vi "Next.vi"(7 "Previous In":refnum<class "Known Host.lvclass">, 8 "Error In":errorcluster, 10 "Next In":refnum<class "Known Host.lvclass">, 11 "KnownHosts In":refnum<class "Known Hosts.lvclass">) -> (0 "Error Out":errorcluster, 1 "Result":T1, 2 "Next Out":refnum<class "Known Host.lvclass">, 3 "KnownHosts Out":refnum<class "Known Hosts.lvclass">, 5 "Previous Out":refnum<class "Known Host.lvclass">)   [LabVIEW 2018, in "Toolkit.lvlib" / "Known Hosts.lvclass"]
uses:
  Known Hosts.lvclass
  Known Host/Known Host.lvclass
  Typedefs/Get Results.ctl
  Known Hosts.lvclass/Known Hosts.ctl
  Known Host/Known Host.lvclass/Known Host.ctl
  Session/Session.lvclass/Session.ctl
  SSH/SSH.lvclass/SSH.ctl
  Toolkit.lvlib
  Session/Session.lvclass
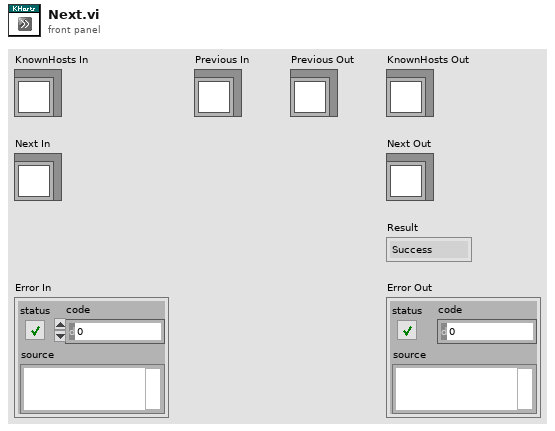
[diagram p1: front panel]
types:
  T1 = typedef "Toolkit.lvlib/Known Hosts.lvclass/Get Results.ctl" = enum32{"Success", "End of Hosts"}
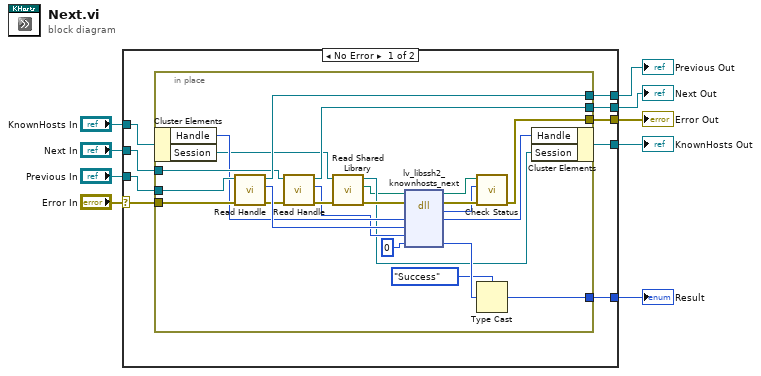
[diagram p0: block diagram]
diagram:
  n1 = case shown="No Error" "Error In" {
    selector: "Error In" -> [w17 w45]
    tunnel: "KnownHosts In" -> [w18 w44]
    tunnel: [w16 w45] -> w7
    tunnel: [w10 w44] -> w6
    tunnel: "Previous In" -> [w15 w43]
    tunnel: [w14 w43] -> w4
    tunnel: [w13 _] -> w3
    tunnel: "Next In" -> [w12 w42]
    tunnel: [w11 w42] -> w1
    frame No Error {
      n2 = in-place {
        in-place-border: w17 -> [w35]
        in-place-border: [w38] -> w16
        in-place-border: w15 -> [w36]
        in-place-border: [w33] -> w14
        in-place-border: [w29] -> w13
        in-place-border: w12 -> [w27]
        in-place-border: [w26] -> w11
        n3 = in-place-cluster #1(w18) -> ("Handle"=w25:u64, "Session"=w21:refnum<class "Session.lvclass">)
        n4 = call "Read Handle.vi"("Error In"=w35, "Known Host In"=w36) -> ("Error Out"=w28:errorcluster, "Handle"=w34:u64, "Known Host Out"=w33:refnum<class "Known Host.lvclass">)  [unwired: 7 in]
        n5 = call "Read Handle.vi"("Error In"=w28, "Known Host In"=w27) -> ("Error Out"=w24:errorcluster, "Handle"=w23:u64, "Known Host Out"=w26:refnum<class "Known Host.lvclass">)  [unwired: 7 in]
        n6 = call "Read Shared Library.vi"("Error In"=w24, "Session In"=w21) -> ("Erorr Out"=w22:errorcluster, "libssh2lv Shared Library"=w19:path, "Session Out"=w20:refnum<class "Session.lvclass">)  [unwired: 7 in]
        n7 = dll-call lib="lv-libssh2.*" fn="lv_libssh2_knownhosts_next"(path in=w19, error in=w22, "handle"=w25, "previous"=w34, "next"=w23, "result"=0) -> (path out=w39:path, error out=w40:errorcluster, "status"=w37:i32, "handle"=w41:u64, "result"=w31:i32)  [unwired: 3 in]
        n8 = call "Check Status.vi"("Error In"=w40, "Status"=w37, "lv-libssh2 Shared Library In"=w39) -> ("Error Out"=w38:errorcluster)  [unwired: 7 in, 1 out]
        n9 = Type Cast(type=Get_Results."Success" ("Get Result"), x=w31) -> (*(type *) &x=w29:T1)
        n10 = in-place-cluster #1("Handle"=w41, "Session"=w20) -> (w10:refnum<class "Known Hosts.lvclass">)
      }
    }
    frame Error {
    }
  }
  "Error Out" <- w7
  "KnownHosts Out" <- w6
  "Previous Out" <- w4
  "Result" <- w3
  "Next Out" <- w1
